vi "S2C_XML_Error.vi"(8 "Error In":errorcluster) -> (0 "Error Out":errorcluster)   [LabVIEW 2015]
uses:
  S2C_XML_Globals.vi
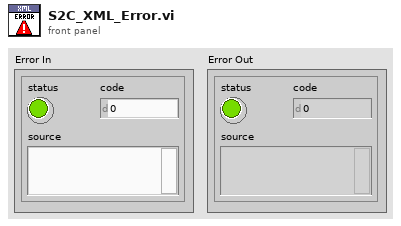
[diagram p1: front panel]
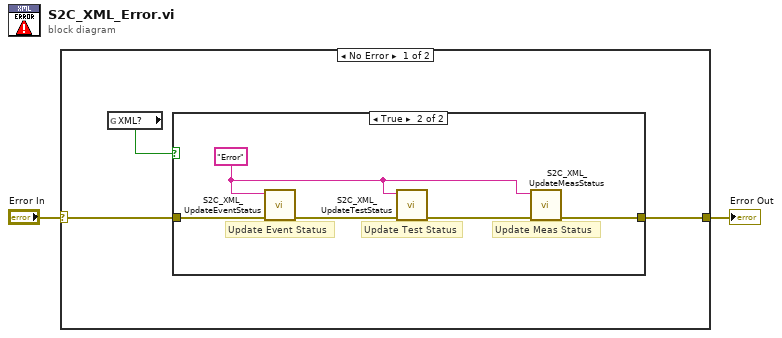
[diagram p0: block diagram]
diagram:
  n1 = case shown="No Error" "Error In" {
    selector: "Error In" -> [w4 w12]
    tunnel: [w5 w12] -> w1
    frame No Error {
      n2 = global read "S2C_XML_Globals.vi" "XML?"() -> (w3:bool)
      n3 = case shown="True" w3 {
        tunnel: [w6 w9] -> w5
        tunnel: w4 -> [w6 w7]
        frame False {
        }
        frame True {
          w8 = "Error"
          # "Update Meas Status"
          # "Update Test Status"
          # "Update Event Status"
          n4 = call "S2C_XML_UpdateEventStatus.vi"("Error In"=w7, "Value"=w8) -> ("Error Out"=w11:errorcluster)  [unwired: 9 in]
          n5 = call "S2C_XML_UpdateTestStatus.vi"("Error In"=w11, "Result"=w8) -> ("Error Out"=w10:errorcluster)  [unwired: 9 in]
          n6 = call "S2C_XML_UpdateMeasStatus.vi"("Error In"=w10, "Result"=w8) -> ("Error Out"=w9:errorcluster)  [unwired: 9 in]
        }
      }
    }
    frame Error {
    }
  }
  "Error Out" <- w1
